vi "Stream Status.vi"(8 "error in (no error)":errorcluster, 11 "RGetStreamStatus in":refnum<class "RGetStreamStatus.lvclass">) -> (0 "error out":errorcluster, 2 "Stream Status":T1, 3 "RGetStreamStatus out":refnum<class "RGetStreamStatus.lvclass">)   [LabVIEW 2022 SP3, in "obs-websocket-lv.lvlib" / "RGetStreamStatus.lvclass"]
uses:
  RGetStreamStatus.lvclass
  RGetStreamStatus.lvclass/RGetStreamStatus.ctl
  Stream Status.ctl
  obs-websocket-lv.lvlib
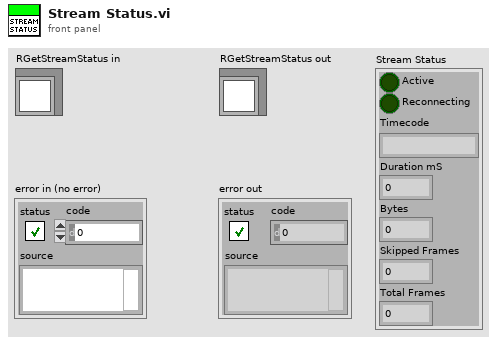
[diagram p1: front panel]
types:
  T1 = typedef "obs-websocket-lv.lvlib/Stream Status.ctl" = cluster{"Active":bool, "Reconnecting":bool, "Timecode":string, "Duration mS":u32, "Bytes":u32, "Skipped Frames":u32, "Total Frames":u32}
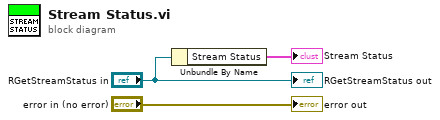
[diagram p0: block diagram]
diagram:
  n1 = Unbundle By Name("RGetStreamStatus in") -> ("Stream Status"=→"Stream Status":T1)
  "error out" <- "error in (no error)"
  "RGetStreamStatus out" <- "RGetStreamStatus in"
